vi "Read TCP Message.vi"(7 "Timeout ms (100)":i32=100, 8 "error in (no error)":errorcluster, 11 "TCP Process in":refnum<class "TCP Process.lvclass">) -> (0 "error out":errorcluster, 1 "Timed out?":bool, 2 "data out":string, 3 "TCP Process out":refnum<class "TCP Process.lvclass">)   [LabVIEW 2019, in "TimingDRV Engine.lvlib" / "TCP Process.lvclass"]
uses:
  TCP Process.lvclass
  TCP Process.lvclass/TCP Process.ctl
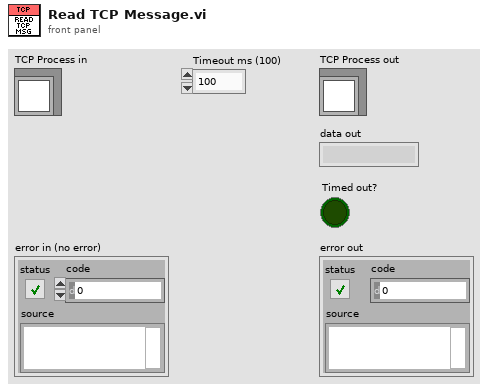
[diagram p1: front panel]
types:
  T1 = enum16{"Standard", "Buffered", "CRLF", "Immediate"}
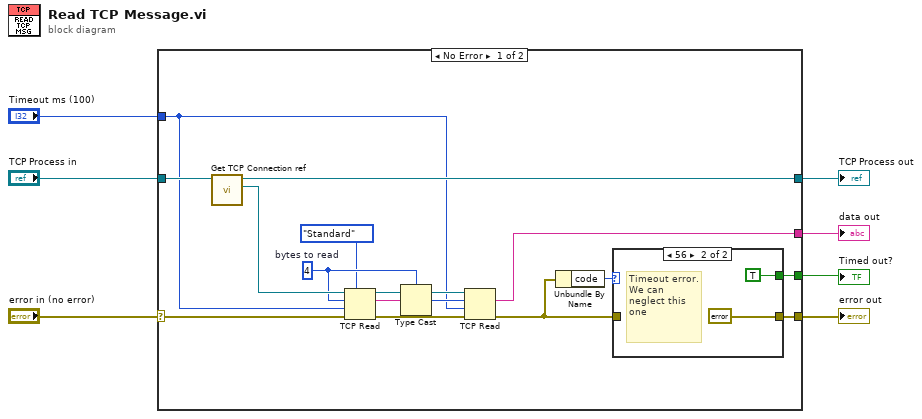
[diagram p0: block diagram]
diagram:
  n1 = case shown="No Error" "error in (no error)" {
    selector: "error in (no error)" -> [w15 w27]
    tunnel: [w10 w27] -> w7
    tunnel: [w23 w28] -> w6
    tunnel: "TCP Process in" -> [w16 w28]
    tunnel: [w14 _] -> w3
    tunnel: "Timeout ms (100)" -> [w13 _]
    tunnel: [w9 _] -> w1
    frame No Error {
      w18 = 4  # bytes to read
      n2 = call "Get TCP Connection ref.vi"("TCP Process in"=w16) -> ("TCP Connection ref"=w19:refnum<k5>, "TCP Process out"=w23:refnum<class "TCP Process.lvclass">)  [unwired: 9 in]
      n3 = TCP Read(connection ID=w19, bytes to read=w18, error in (no error)=w15, 7:T1."Standard" ("mode (standard)"), 9:w13) -> (connection ID out=w22:refnum<k5>, data out=w17:string, error out=w20:errorcluster)
      n4 = Type Cast(type=w18, x=w17) -> (*(type *) &x=w21:i32)
      n5 = TCP Read(connection ID=w22, bytes to read=w21, error in (no error)=w20, 9:w13) -> (data out=w14:string, error out=w11:errorcluster)  [unwired: 1 in, 1 out]
      n6 = Unbundle By Name(w11) -> ("code"=w12:i32)
      n7 = case shown="56" w12 {
        tunnel: w11 -> [w24 _]
        tunnel: [w24 errorcluster {"status"=FALSE, "code"=0, "source"=""} ("error out")] -> w10
        tunnel: [_ TRUE ("Timed out?")] -> w9
        frame 0, Default {
        }
        frame 56 {
          # "Timeout error. We can neglect this one"
        }
      }
    }
    frame Error {
    }
  }
  "error out" <- w7
  "TCP Process out" <- w6
  "data out" <- w3
  "Timed out?" <- w1
